vi "获取指令字节.vi"(8 "字符串":string, 11 "字节数":i32) -> (1 "指令":string, 2 "16进制字符串":string)   [LabVIEW 2016]
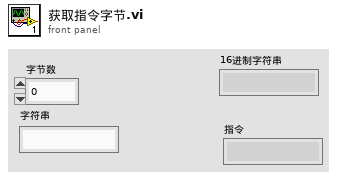
[diagram p1: front panel]
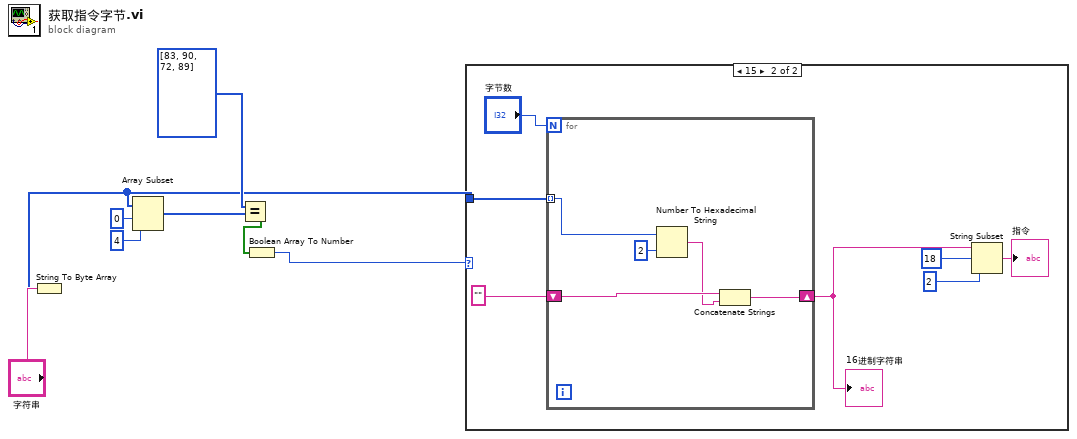
[diagram p0: block diagram]
diagram:
  n1 = String To Byte Array(string="字符串") -> (unsigned byte array=w1:u8[])
  n2 = Array Subset(array=w1, index=0 ("索引"), length=4 ("长度")) -> (w4:u8[])
  n3 = Equal?(x=u8[] [83, 90, 72, 89], y=w4) -> (x = y?=w5:bool[])
  n4 = Boolean Array To Number(Boolean array=w5) -> (number=w3:u32)
  n5 = case shown="15" w3 {
    tunnel: w1 -> [_ w15]
    frame 0, Default {
    }
    frame 15 {
      n6 = for {
        N: "字节数" -> [_]
        tunnel: w15 -> [w19] mode=indexing
        shift-right: [w16] -> w11
        shift-left: "" -> [w18]
        n7 = Number To Hexadecimal String(1:i16 2 ("宽度(-)"), 2:w19) -> (0:w17:string)
        n8 = Concatenate Strings(w18, w17) -> (w16:string)
      }
      "16进制字符串" <- w11
      n9 = String Subset(string=w11, offset (0)=18 ("偏移量(0)"), length (rest)=2 ("长度（剩余）")) -> (substring=→"指令":string)
    }
  }
